vi "Write_PZT_File.vi"(8 "error in":errorcluster, 10 "Layer Data":T1[](array[typedef]), 11 "PZT filename":path) -> (0 "error out":errorcluster)   [LabVIEW 2022 SP3]
uses:
  Custom_Piezo.ctl
  PZT type.ctl
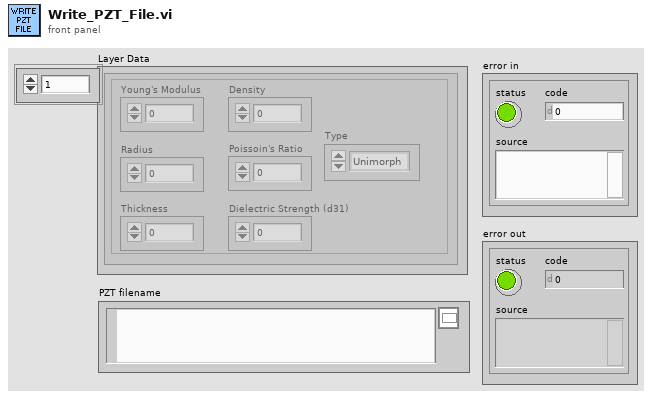
[diagram p1: front panel]
types:
  T1 = typedef "Custom_Piezo.ctl" = cluster{"Young's Modulus":dbl, "Radius":dbl, "Density":dbl, "Poissoin's Ratio":dbl, "Thickness":dbl, "Dielectric Strength (d31)":dbl, "Type":T2}
  T2 = typedef "PZT type.ctl" = enum16{"Bimorph", "Unimorph"}
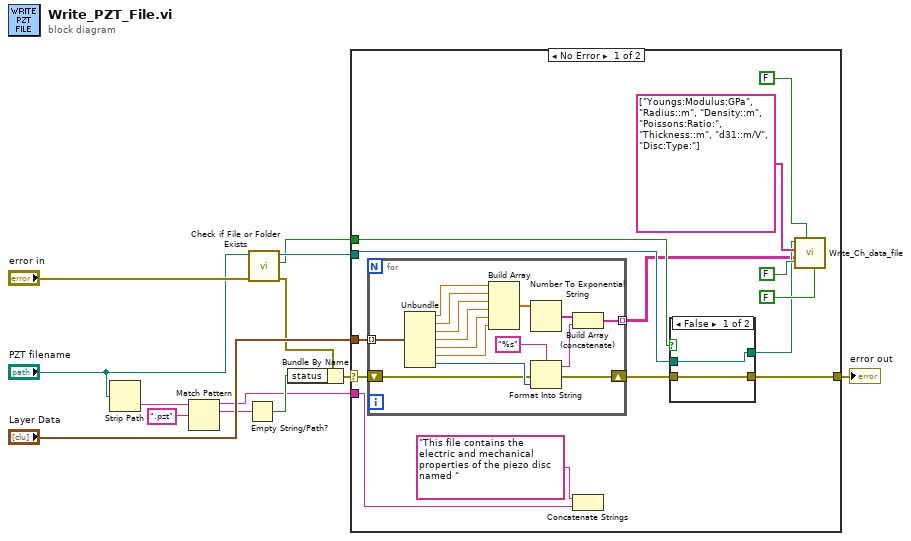
[diagram p0: block diagram]
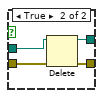
[diagram p2: hidden frame]
diagram:
  n1 = Strip Path(path="PZT filename") -> (name=w10:string)  [unwired: 1 out]
  n2 = Match Pattern(string=w10, regular expression=".pzt") -> (before substring=w3:string, match substring=w8:string)  [unwired: 1 in, 2 out]
  n3 = Empty String/Path?(string/path=w8) -> (empty?=w7:bool)
  n4 = call <vilib>:"Check if File or Folder Exists.vi"("error in (no error)"="error in", "path"="PZT filename") -> ("error out"=w4:errorcluster, "file or folder exists?"=w11:bool, "dup path"=w12:path)  [unwired: 7 in]
  n5 = Bundle By Name(cluster=w4, "status"=w7) -> (w6:errorcluster)
  n6 = case shown="No Error" w6 {
    selector: w6 -> [w18 w49]
    tunnel: "Layer Data" -> [w27 _]
    tunnel: w12 -> [w22 _]
    tunnel: w11 -> [w21 _]
    tunnel: w3 -> [w20 _]
    tunnel: [w16 w49] -> w2
    frame No Error {
      n7 = for {
        tunnel: w27 -> [w48] mode=indexing
        tunnel: [w36] -> w15 mode=indexing
        shift-right: [w34] -> w17
        shift-left: w18 -> [w35]
        n8 = Unbundle(w48) -> ("Young's Modulus"=w47:dbl, "Radius"=w46:dbl, "Density"=w45:dbl, "Poissoin's Ratio"=w44:dbl, "Thickness"=w43:dbl, "Dielectric Strength (d31)"=w42:dbl, "Type"=w39:T2)
        n9 = Build Array(w47, w46, w45, w44, w43, w42) -> (w41:dbl[])
        n10 = Number To Exponential String(number=w41) -> (E-format string=w40:string[])  [unwired: 3 in]
        n11 = Format Into String(format string="%s", error in=w35, w39) -> (resulting string=w37:string, error out=w34:errorcluster)  [unwired: 1 in]
        n12 = Build Array (concatenate)(w40, w37) -> (w36:string[])
      }
      n13 = Concatenate Strings("This file contains the electric and mechanical properties of the piezo disc named " ("string"), w20) -> ()  [unwired: 1 out]
      n14 = case shown="False" w21 {
        tunnel: [w29 w32] -> w23
        tunnel: w22 -> [w29 w33]
        tunnel: w17 -> [w28 w31]
        tunnel: [w28 w30] -> w16
        frame False {
        }
        frame True {
          n15 = Delete(path (use dialog)=w33, error in=w31) -> (deleted path=w32:path, error out=w30:errorcluster)  [unwired: 3 in, 1 out]
        }
      }
      n16 = call "Write_Ch_data_file.vi"("Append last row only"=FALSE, 6:FALSE ("append to file? (new file:F)"), "exists?"=FALSE, "Channel Values"=w15, "Channel names"=string[] ["Youngs:Modulus:GPa", "Radius::m", "Density::m", "Poissons:Ratio:", "Thickness::m", "d31::m/V", "Disc:Type:"], "Filename"=w23) -> ()  [unwired: 2 in, 4 out]
    }
    frame Error {
    }
  }
  "error out" <- w2
